vi "Untitled 3.vi"() -> ()   [LabVIEW 2020]
uses:
  <vilib>/Analysis/baseanly.llb/Mean (DBL).vi
  <vilib>/Analysis/NI_AALBase.lvlib
panel:
  out "数据":dbl[][](array[numeric])
  in  "电压上限（V）":dbl
  in  "电压递增步长（V）":dbl
  in  "采集时间间隔":dbl[unit]
  in  "标准电阻值（欧姆）":dbl
  in  "开关":bool
  out "XY Graph":cluster{"Y":dbl[], "Y":dbl[]}[](graph)
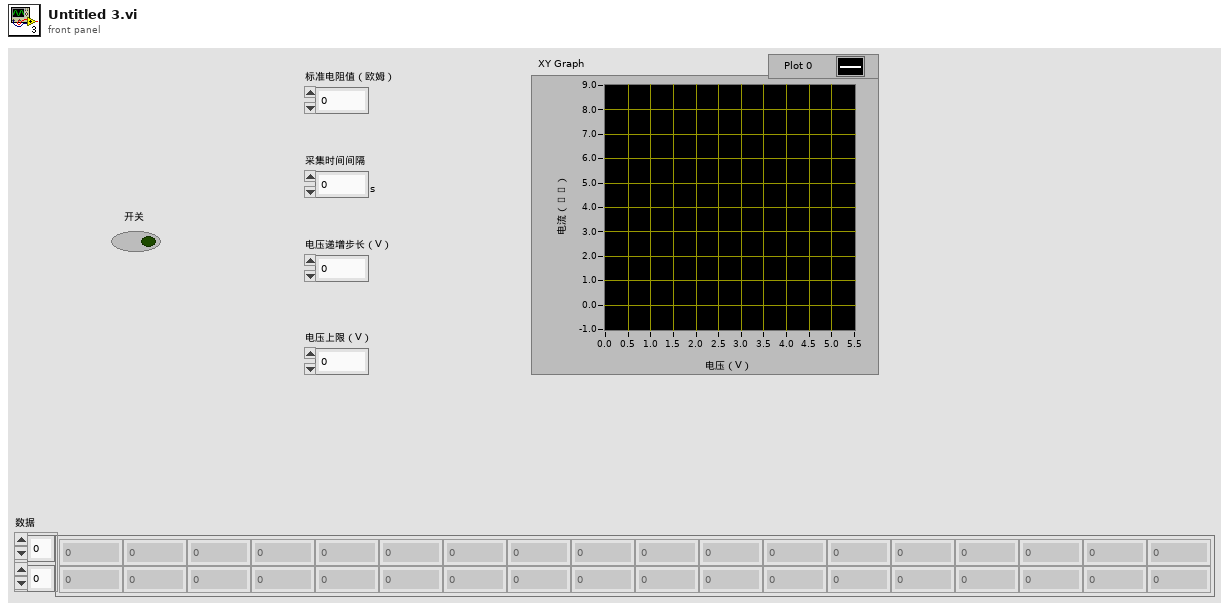
[diagram p1: front panel]
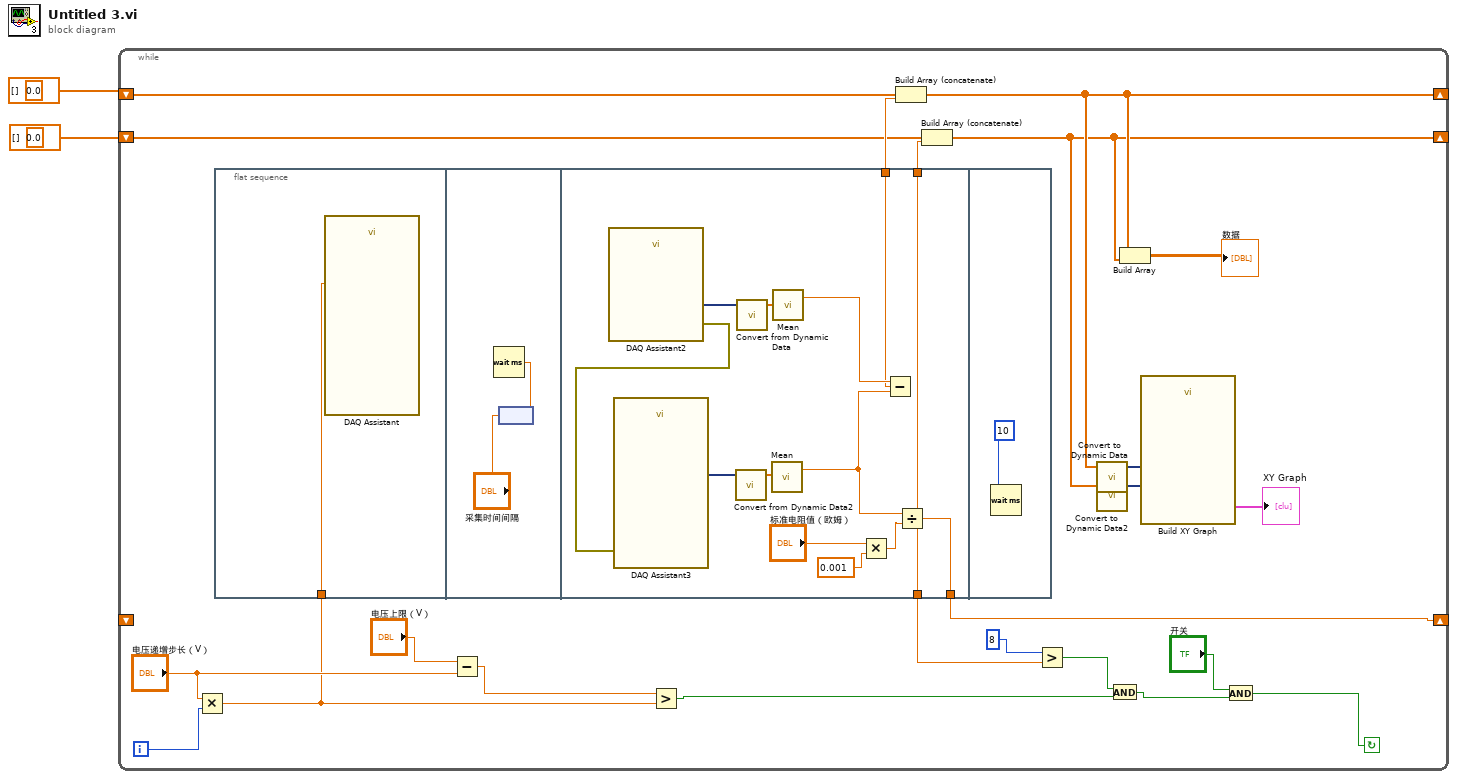
[diagram p0: block diagram]
diagram:
  (unwired) 0.0 ("element")
  (unwired) 0.0 ("element")
  n1 = while {
    shift-right: [w17] -> _
    shift-left: dbl[] [] ("appended array") -> [w22]
    shift-right: [w19] -> _
    shift-left: dbl[] [] ("appended array") -> [w24]
    shift-right: [w14] -> _
    shift-left: _ -> [_]
    i -> [w25]
    stop <- w3 continue-if-true
    n2 = Multiply(x="电压递增步长（V）", y=w25) -> (x*y=w9:dbl)
    n3 = flat-sequence {
      tunnel: w9 -> [w26]
      tunnel: [w33] -> w23
      tunnel: [w29] -> w21
      tunnel: [w29] -> w14
      tunnel: [w29] -> w13
      frame #0 {
        n4 = call "DAQ Assistant"("data"=w26) -> ()  [unwired: 17 in, 2 out]
      }
      frame #1 {
        n5 = node("采集时间间隔") -> (w28:dbl)
        n6 = Wait (ms)(milliseconds to wait=w28) -> ()  [unwired: 1 out]
      }
      frame #2 {
        n7 = call "DAQ Assistant2"() -> ("data"=w39:dynamicdata, "error out"=w40:errorcluster)  [unwired: 17 in, 1 out]
        n8 = call "DAQ Assistant3"("error in"=w40) -> ("data"=w37:dynamicdata)  [unwired: 16 in, 2 out]
        n9 = call "Convert from Dynamic Data2"("Dynamic Data Type"=w37) -> ("Array"=w36:dbl[])  [unwired: 3 in]
        n10 = call "Convert from Dynamic Data"("Dynamic Data Type"=w39) -> ("Array"=w38:dbl[])  [unwired: 3 in]
        n11 = call-poly <vilib>:"Mean.vi"("X"=w36) -> ("mean"=w34:dbl)  [unwired: 1 out]
        n12 = call-poly <vilib>:"Mean.vi"("X"=w38) -> ("mean"=w35:dbl)  [unwired: 1 out]
        n13 = Multiply(x="标准电阻值（欧姆）", y=0.001) -> (x*y=w30:dbl)
        n14 = Subtract(x=w35, y=w34) -> (x-y=w33:dbl)
        n15 = Divide(x=w34, y=w30) -> (x/y=w29:dbl)
      }
      frame #3 {
        n16 = Wait (ms)(milliseconds to wait=10) -> ()  [unwired: 1 out]
      }
    }
    n17 = Subtract(x="电压上限（V）", y="电压递增步长（V）") -> (x-y=w10:dbl)
    n18 = Greater?(x=w10, y=w9) -> (0:w8:bool)
    n19 = Build Array (concatenate)(w24, w23) -> (w19:dbl[])
    n20 = Build Array (concatenate)(w22, w21) -> (w17:dbl[])
    n21 = Greater?(x=8, y=w13) -> (0:w6:bool)
    n22 = call "Convert to Dynamic Data"("Array"=w19) -> ("Dynamic Data Type"=w18:dynamicdata)  [unwired: 3 in]
    n23 = call "Convert to Dynamic Data2"("Array"=w17) -> ("Dynamic Data Type"=w16:dynamicdata)  [unwired: 3 in]
    n24 = And(x=w6, y=w8) -> (x .and. y?=w4:bool)
    n25 = Build Array(w19, w17) -> (→"数据":dbl[][])
    n26 = call "Build XY Graph"("Y Input"=w16, "X Input"=w18) -> ("XY Graph"=→"XY Graph":cluster{"X":dbl[], "Y":dbl[]}[])  [unwired: 8 in, 1 out]
    n27 = And(x="开关", y=w4) -> (x .and. y?=w3:bool)
  }
